vi "Wave_to_SFTF_Batch.vi"(6 "Img. Res.":i32=150, 7 "STFT Config":T1={"FFT block size"=1024, "window"=3, "time segment"={"from [s]"=-1.0, "to [s]"=-1.0, "time increment"=20.645, "time increment units (%)"=enum."%"}, "dB On (T)"=TRUE, "Dynamic Range(dB)"=80.0, "Mel?"=TRUE} {"window" items=["None "=0, "Hanning"=1, "Hamming"=2, "Blackman-Harris"=3, "Exact Blackman"=4, "Blackman"=5, "Flat Top"=6, "4 Term B-Harris "=7, "7 Term B-Harris"=8, "Low Sidelobe"=9, "Blackman Nuttall"=11]}, 8 "error in (no error)":errorcluster, 10 "path to dest.":path, 11 "path to wav":path=path "D:/DNN/data/Sound/30words/train/audio/bed") -> (0 "error out":errorcluster)   [LabVIEW 2020]
uses:
  Controls/Wave2STFT_Cfg.ctl
  <vilib>/vision/NI_Vision_Development_Module.lvlib
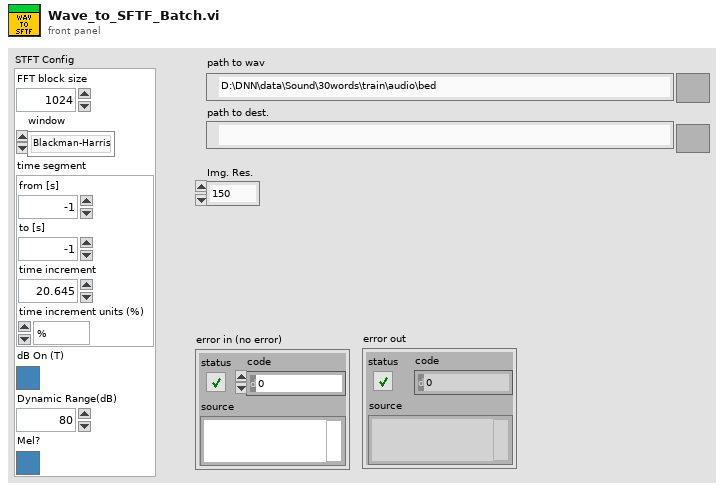
[diagram p1: front panel]
types:
  T1 = typedef "Wave2STFT_Cfg.ctl" = cluster{"FFT block size":i32, "window":u16, "time segment":cluster{"from [s]":dbl, "to [s]":dbl, "time increment":dbl, "time increment units (%)":enum16{"%", "s", "ms"}}, "dB On (T)":bool, "Dynamic Range(dB)":sgl, "Mel?":bool}
  T2 = typedef "Image Type" = u32
  T3 = typedef "IMAQ Image.ctl" = refnum<image>
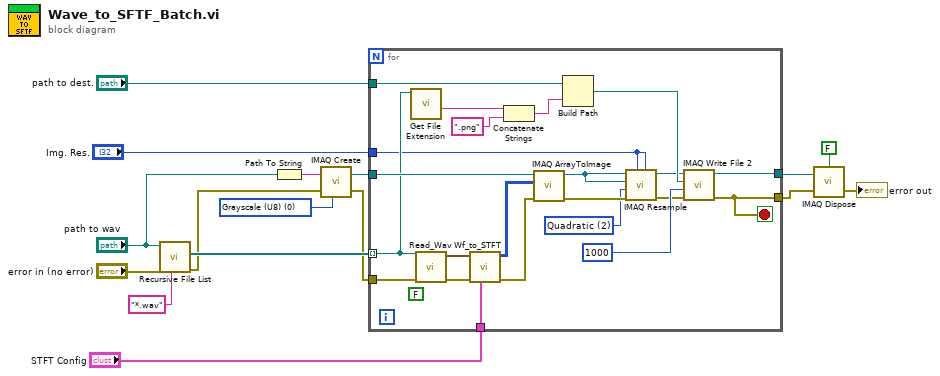
[diagram p0: block diagram]
diagram:
  w7 = T2 0 items=["Grayscale (U8)", "Grayscale (I16)", "Grayscale (SGL)", "Complex (CSG)", "RGB (U32)", "HSL (U32)", "RGB (U64)", "Grayscale (U16)"] ("Image Type")
  n1 = call <vilib>:"Recursive File List.vi"("pattern"="*.wav", "error in (no error)"="error in (no error)", "Folder Path"="path to wav") -> ("error out"=w6:errorcluster, "All Files in Dir"=w11:path[])  [unwired: 4 in, 3 out]
  n2 = Path To String(path="path to wav") -> (string=w8:string)
  n3 = call "IMAQ Create"("Image Name"=w8, "Image Type"=w7, "error in (no error)"=w6) -> ("New Image"=w16:T3, "error out"=w5:errorcluster)  [unwired: 2 in]
  n4 = for {
    tunnel: w11 -> [w31] mode=indexing
    tunnel: w16 -> [w37]
    tunnel: [w38] -> w15
    tunnel: [w30] -> w14
    tunnel: w5 -> [w36]
    tunnel: "path to dest." -> [w35]
    tunnel: "STFT Config" -> [w18]
    tunnel: "Img. Res." -> [w17]
    stop <- w30 stop-if-true
    w20 = u32 2 items=["Zero Order", "Bi-Linear", "Quadratic", "Cubic Spline"] ("Interpolation Type")
    (unwired) FALSE ("align?")
    n5 = call <vilib>:"Get File Extension.vi"("file"=w31) -> ("filename without extension"=w32:string)  [unwired: 6 in, 4 out]
    n6 = call "Read_Wav.vi"("error in (no error)"=w36, "Path to wav"=w31) -> ("error out"=w34:errorcluster, "wf"=w33:waveform(dbl))  [unwired: 8 in]
    n7 = call "Wf_to_STFT.vi"("STFT Config"=w18, "error in (no error)"=w34, "WF"=w33) -> ("error out"=w25:errorcluster, "Image_data"=w27:u8[][])  [unwired: 6 in, 1 out]
    n8 = Concatenate Strings(w32, ".png" ("name or relative path")) -> (w23:string)
    n9 = call "IMAQ ArrayToImage"("error in (no error)"=w25, "Image Pixels (U8)"=w27, "Image"=w37) -> ("error out"=w28:errorcluster, "Image Out"=w29:T3)  [unwired: 7 in]
    n10 = Build Path(base path=w35, name or relative path=w23) -> (appended path=w24:path)
    n11 = call "IMAQ Resample"("X Resolution"=w17, "Y Resolution"=w17, "error in (no error)"=w28, "Interpolation Type"=w20, "Image Dst"=w29, "Image Src"=w29) -> ("error out"=w19:errorcluster, "Image Dst Out"=w22:T3)  [unwired: 4 in]
    n12 = call-poly "IMAQ Write File 2"("error in (no error)"=w19, "Image Quality"=u32 1000, "File Path"=w24, "Image"=w22) -> ("error out"=w30:errorcluster, "Image Out (duplicate)"=w38:T3)  [unwired: 6 in]
  }
  n13 = call "IMAQ Dispose"("All Images? (No)"=FALSE, "Image"=w15, "error in (no error)"=w14) -> ("error out"=→"error out":errorcluster)  [unwired: 3 in]
